vi "Read-from-file-by-reference.vi"(8 "error in (no error)":errorcluster, 9 "Update values?":bool, 10 "Controls by reference":refnum<vi>[](array[refnum]), 11 "SettingsFile in":refnum<class "SettingsFile.lvclass">) -> (0 "error out":errorcluster, 2 "Values":T1(array[cluster]), 3 "SettingsFile out":refnum<class "SettingsFile.lvclass">)   [LabVIEW 2013, in "SettingsFile.lvlib" / "SettingsFile.lvclass"]
uses:
  SettingsFile.lvclass
  SettingsFile.lvclass/SettingsFile.ctl
  <vilib>/Utility/config.llb/Config Data RefNum.ctl
  Errors.ctl
  <vilib>/Utility/xml.llb/Read From XML File(string).vi
  <vilib>/Utility/config.llb/Read Key (String).vi
  <vilib>/Utility/config.llb/NI_LVConfig.lvlib
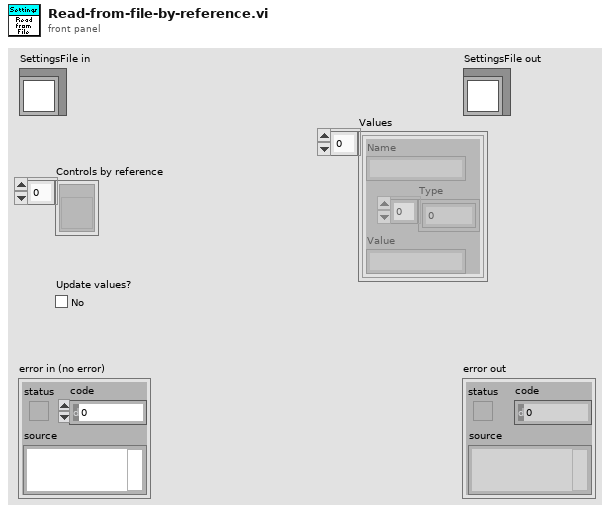
[diagram p1: front panel]
types:
  T1 = cluster{"Name":string, "Type":i16[], "Value":string}[]
  T2 = typedef "NI_LVConfig.lvlib/Config Data RefNum.ctl" = refnum<k1>
  T3 = cluster{"Name":string, "Type":i16[], "Value":string}
  T4 = typedef "SettingsFile.lvlib/SettingsFile.lvclass/Errors.ctl" = enum16{"Not implemented", "Command not recognized", "Invalid input", "No connection", "Timeout", "Invalid file type", "No file access"}
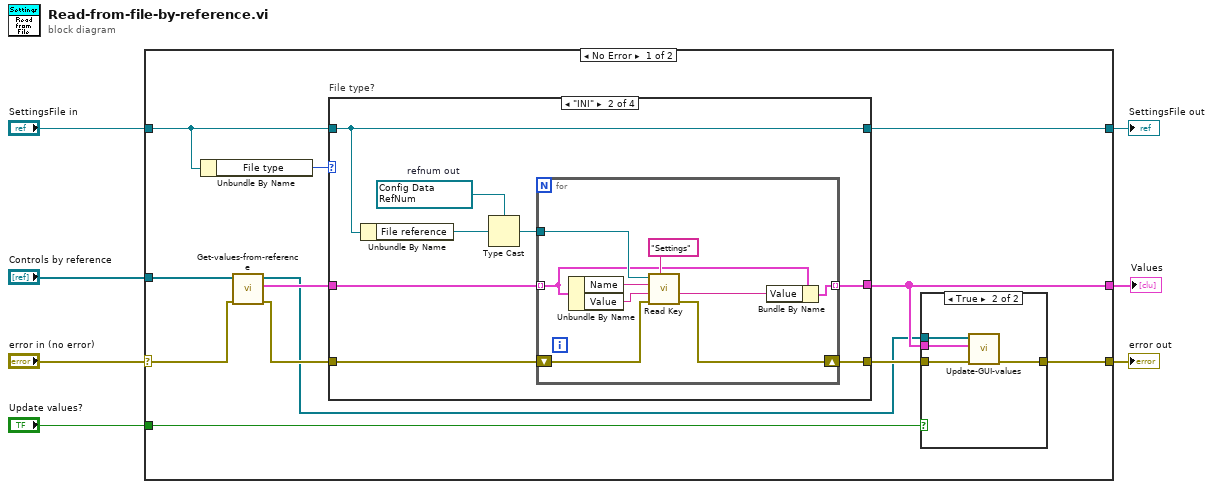
[diagram p0: block diagram]
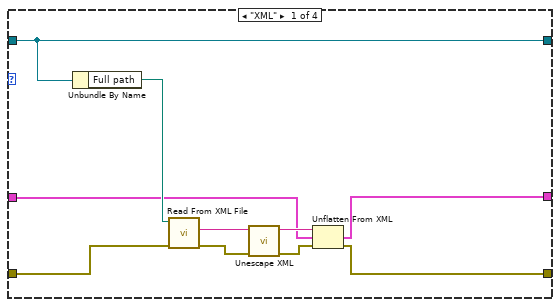
[diagram p3: hidden frame]
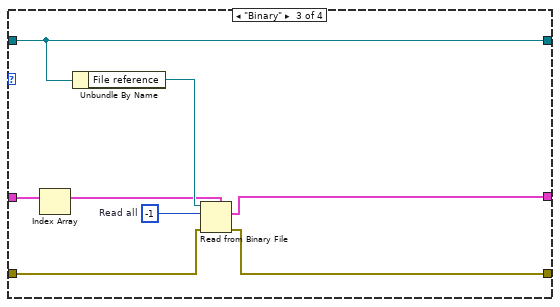
[diagram p4: hidden frame]
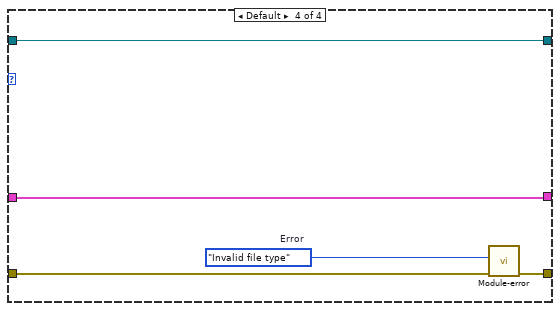
[diagram p5: hidden frame]
diagram:
  n1 = case shown="No Error" "error in (no error)" {
    selector: "error in (no error)" -> [w15 w66]
    tunnel: [w11 w66] -> w6
    tunnel: [w17 w65] -> w4
    tunnel: "SettingsFile in" -> [w18 w65]
    tunnel: "Controls by reference" -> [w16 _]
    tunnel: "Update values?" -> [w8 _]
    tunnel: [w10 _] -> w1
    frame No Error {
      n2 = Unbundle By Name(w18) -> ("File type"=w19:enum16{"XML", "INI", "Binary"})
      n3 = call "Get-values-from-reference.vi"("error in (no error)"=w15, "Controls to save in"=w16) -> ("error out"=w14:errorcluster, "Values"=w13:T1, "Controls to save out"=w9:refnum<vi>[])  [unwired: 7 in]
      n4 = case "File type?" shown="\"INI\"" w19 {
        tunnel: w18 -> [w33 w42 w59 w64]
        tunnel: [w33 w42 w59 w64] -> w17
        tunnel: w14 -> [w32 w40 w57 w62]
        tunnel: [w25 w41 w56 w63] -> w12
        tunnel: w13 -> [w27 w36 w54 w60]
        tunnel: [w26 w35 w53 w60] -> w10
        frame "XML" {
          n5 = Unbundle By Name(w33) -> ("Full path"=w34:path)
          n6 = call-poly <vilib>:"Read From XML File.vi"("error in (no error)"=w32, "XML File Path"=w34) -> ("error out"=w31:errorcluster, "XML Elements"=w30:string)  [unwired: 7 in, 1 out]
          n7 = call <vilib>:"Unescape XML.vi"("error in (no error)"=w31, "XML String In"=w30) -> ("error out"=w29:errorcluster, "XML String Out"=w28:string)  [unwired: 8 in]
          n8 = Unflatten From XML(xml string=w28, type=w27, error in (no error)=w29) -> (value=w26:T1, error out=w25:errorcluster)
        }
        frame "INI" {
          w39 = T2 refnum items=["config data"]  # refnum out
          n9 = Unbundle By Name(w42) -> ("File reference"=w38:refnum<file>)
          n10 = Type Cast(type=w39, x=w38) -> (*(type *) &x=w37:T2)
          n11 = for {
            shift-right: [w50] -> w41
            shift-left: w40 -> [w51]
            tunnel: w37 -> [w46]
            tunnel: w36 -> [w45] mode=indexing
            tunnel: [w43] -> w35 mode=indexing
            n12 = Unbundle By Name(w45) -> ("Name"=w48:string, "Value"=w47:string)
            n13 = call-poly <vilib>:"Read Key.vi"("section"="Settings", "error in (no error)"=w51, "default value"=w47, "key"=w48, "refnum"=w46) -> ("error out"=w50:errorcluster, "value"=w44:string)  [unwired: 3 in, 2 out]
            n14 = Bundle By Name(cluster=w45, "Value"=w44) -> (w43:T3)
          }
        }
        frame "Binary" {
          w55 = -1  # Read all
          n15 = Index Array(array=w54) -> (element=w52:T3)  [unwired: 1 in]
          n16 = Unbundle By Name(w59) -> ("File reference"=w58:refnum<file>)
          n17 = Read from Binary File(5:w52, 8:w57, 10:w55, 11:w58) -> (0:w56:errorcluster, 2:w53:T1)  [unwired: 2 in, 2 out]
        }
        frame Default {
          w61 = Errors."Invalid file type"  # Error
          n18 = call "Module-error.vi"("error in (no error)"=w62, "Error"=w61) -> ("error out"=w63:errorcluster)  [unwired: 9 in]
        }
      }
      n19 = case shown="True" w8 {
        tunnel: w12 -> [w20 w24]
        tunnel: [w20 w23] -> w11
        tunnel: w10 -> [_ w22]
        tunnel: w9 -> [_ w21]
        frame False {
        }
        frame True {
          n20 = call "Update-GUI-values.vi"("error in (no error)"=w24, "New values"=w22, "Controls in"=w21) -> ("error out"=w23:errorcluster)  [unwired: 6 in, 2 out]
        }
      }
    }
    frame Error {
    }
  }
  "error out" <- w6
  "SettingsFile out" <- w4
  "Values" <- w1
